vi "7HP_Create datalog header string.vi"() -> (0 "Datalog header string":string)   [LabVIEW 2017]
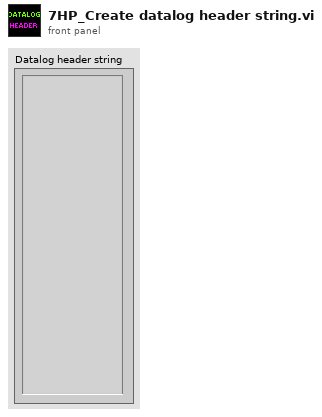
[diagram p1: front panel]
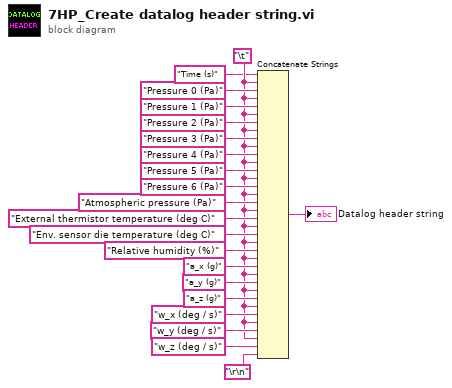
[diagram p0: block diagram]
diagram:
  w2 = "\t"
  n1 = Concatenate Strings("Time (s)", w2, "Pressure 0 (Pa)", w2, "Pressure 1 (Pa)", w2, "Pressure 2 (Pa)", w2, "Pressure 3 (Pa)", w2, "Pressure 4 (Pa)", w2, "Pressure 5 (Pa)", w2, "Pressure 6 (Pa)", w2, "Atmospheric pressure (Pa)", w2, "External thermistor temperature (deg C)", w2, "Env. sensor die temperature (deg C)", w2, "Relative humidity (%)", w2, "a_x (g)", w2, "a_y (g)", w2, "a_z (g)", w2, "w_x (deg / s)", w2, "w_y (deg / s)", w2, "w_z (deg / s)", "\r\n") -> (→"Datalog header string":string)
